vi "Log Message set (SubVI).vi"(10 "Communication":T1(array[cluster]), 11 "Command":T2) -> ()   [LabVIEW 2025]
uses:
  Communication Handle/API/Commands.ctl
  <vilib>/Utility/file.llb/Write Delimited Spreadsheet (string).vi
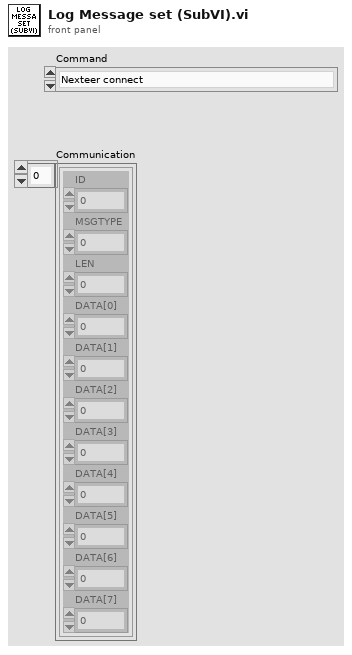
[diagram p1: front panel]
types:
  T1 = cluster{"ID":u32, "MSGTYPE":u8, "LEN":u8, "DATA[0]":u8, "DATA[1]":u8, "DATA[2]":u8, "DATA[3]":u8, "DATA[4]":u8, "DATA[5]":u8, "DATA[6]":u8, "DATA[7]":u8}[]
  T2 = typedef "Commands.ctl" = enum16{"Nexteer connect", "Write Polarity", "Write BEMF", "Write Torque Scale Sensors T1", "Write Torque Scale Sensors T2", "Trim HW Torque Sensors T1", "Trim HW Torque Sensors T2", "Read HW Torque Trim Performed Sensors T1", "Read HW Torque Trim Performed Sensors T2", "Write EOL Offset values to defaults", "Write EOL Gain values to defaults", "Write Serial Number", "Write Hardware Part Number", "Write EPS Serial Number", "Read MEC Counter", "MCU Reset", "Read System State", "Read First Motor Position", "Manufacturing Diagnostic Defeat", "Perform Current Offset ", "Current Offset Status", "Enable Engine Run", "Perform Current Gain ", "Current Gain Status", "Disable Torque Ramp Down ", "Disable Engine Run", "Set Vehicle Speed Override", "Read Offset Values Using FD F5", "Read Gain Values Using FD F4", "Clear Nexteer NTCs", "Read Second Motor Position", "Read ECU Software ID", "Read Internal Software Version", "Read Bootloader ID", "Read Bootloader Software Version", "Read Calibration Release 0", "Read Calibration Release 1", "Read Calibration Release 2", "Read Temperature  ", "Battery Voltage  ", "Read Motor Angle 0", "Read Motor Angle 1 ", "Set Motor Torque Command ", "Read Motor Current   ", "Stop Motor Torque Command", "Read NTCs", "Read Serial Number", "Read HW Part Number", "Read Polarity", "Set NVM Access Defeat", "Read Software Release", "Read Software Build Date", "Write Single Inverter Hardware value", "Write Dual Inverter Hardware value", "Read Single Inverter HW Value", "Read Dual Inverter HW Value", "Write MEC Counter FE", "Write MEC Counter FF", "Read BEMF", "Read Torque 1 FDB6", "Read Torque 2 FDB7", "Read Torque Trim 1 FDB4", "Read Torque Trim 2 FDB5", "Write Torque Trim 1 FDB4", "Write Torque Trim 2 FDB5", "XCP connect", "Read HW Torque T1", "Read HW Torque T2", "Read Motor Speed "}
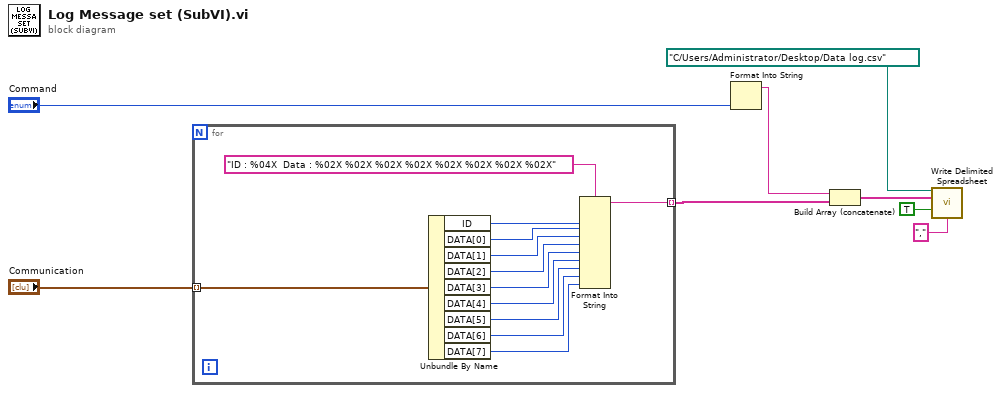
[diagram p0: block diagram]
diagram:
  n1 = for {
    tunnel: "Communication" -> [w20] mode=indexing
    tunnel: [w9] -> w4 mode=indexing
    n2 = Unbundle By Name(w20) -> ("ID"=w19:u32, "DATA[0]"=w18:u8, "DATA[1]"=w17:u8, "DATA[2]"=w16:u8, "DATA[3]"=w15:u8, "DATA[4]"=w14:u8, "DATA[5]"=w13:u8, "DATA[6]"=w12:u8, "DATA[7]"=w11:u8)
    n3 = Format Into String(format string="ID : %04X  Data : %02X %02X %02X %02X %02X %02X %02X %02X", w19, w18, w17, w16, w15, w14, w13, w12, w11) -> (resulting string=w9:string)  [unwired: 2 in, 1 out]
  }
  n4 = Format Into String("Command") -> (resulting string=w3:string)  [unwired: 3 in, 1 out]
  n5 = Build Array (concatenate)(w3, w4) -> (w5:string[])
  n6 = call-poly <vilib>:"Write Delimited Spreadsheet.vi"("file path (dialog if empty)"=path "C:/Users/Administrator/Desktop/Data log.csv", "1D data"=w5, "append to file? (new file:F)"=TRUE, "delimiter (\\t)"="," ("delimiter (\\t)")) -> ()  [unwired: 10 in, 2 out]
